vi "Shutdown FPGA Resource Manager Visualizer.vi"(8 "error in (no error)":errorcluster) -> (0 "error out":errorcluster)   [LabVIEW 2016, in "FPGA RM System Definition API.lvlib"]
uses:
  FPGA RM System Definition API.lvlib
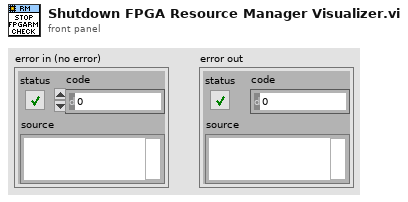
[diagram p1: front panel]
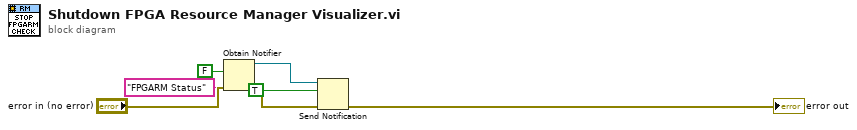
[diagram p0: block diagram]
diagram:
  n1 = Obtain Notifier(name (unnamed)="FPGARM Status", notification data type=FALSE, error in (no error)="error in (no error)") -> (notifier out=w5:refnum<notifier>, error out=w7:errorcluster)  [unwired: 1 in, 1 out]
  n2 = Send Notification(notification=TRUE, notifier=w5, error in (no error)=w7) -> (error out=→"error out":errorcluster)  [unwired: 1 out]
